vi "Fancy Slide Update.vi"(8 "error in (no error)":errorcluster, 11 "Slide in":refnum<vi>) -> (0 "error out":errorcluster)   [LabVIEW 2018]
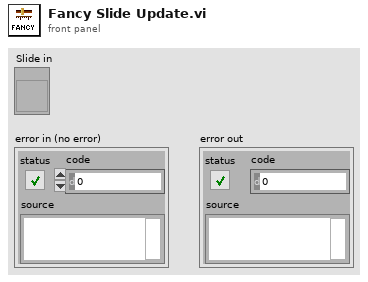
[diagram p1: front panel]
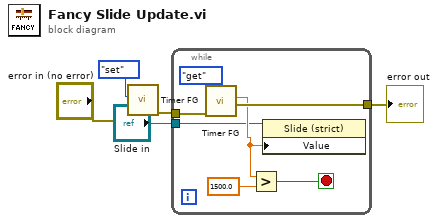
[diagram p0: block diagram]
diagram:
  n1 = call "Timer FG.vi"("error in"="error in (no error)", "Action"=enum16{"set", "get"}."set") -> ("error out"=w5:errorcluster)  [unwired: 8 in, 1 out]
  n2 = while {
    tunnel: w5 -> [w12]
    tunnel: [w9] -> w2
    tunnel: "Slide in" -> [w6]
    stop <- w10 stop-if-true
    n3 = call "Timer FG.vi"("error in"=w12, "Action"=enum16{"set", "get"}."get") -> ("error out"=w9:errorcluster, "Elapsed time (ms)"=w7:dbl)  [unwired: 8 in]
    n4 = Greater?(x=w7, y=1500.0) -> (0:w10:bool)
    n5 = property on="Property Node" class="Slide (strict)"(reference=w6, "Value"=w7) -> ()  [unwired: 1 in, 2 out]
  }
  "error out" <- w2
